vi "Get Active Timing Function.vi"(0 "Timing Functions in":refnum<class "ControllerData.lvclass">, 11 "error in (no error)":errorcluster) -> (4 "Timing Functions out":refnum<class "ControllerData.lvclass">, 6 "Function List":T1, 15 "error out":errorcluster)   [LabVIEW 2019, in "ControllerData.lvclass"]
uses:
  ControllerData.lvclass
  source code/LSL components/functions/functionsbase/functionbase.lvclass
  Function List.ctl
  D:/Pet Projects/LSL/source code/LSL components/functions/functionsbase/functionbase.lvclass
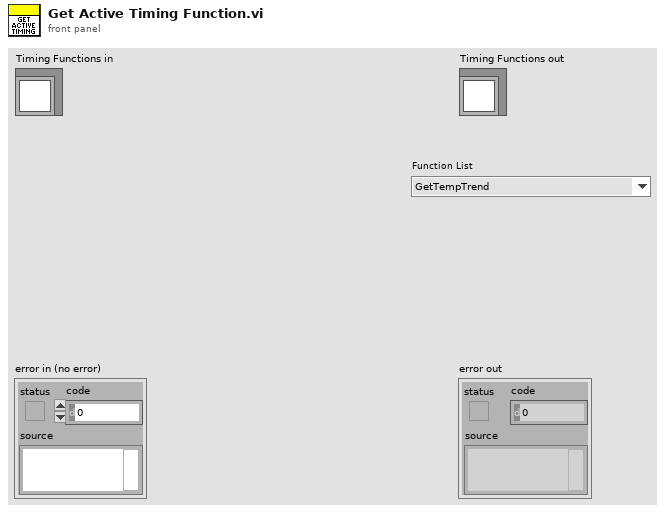
[diagram p1: front panel]
types:
  T1 = typedef "ControllerData.lvclass/Function List.ctl" = enum16{"GetTempTrend", "GetStatus"}
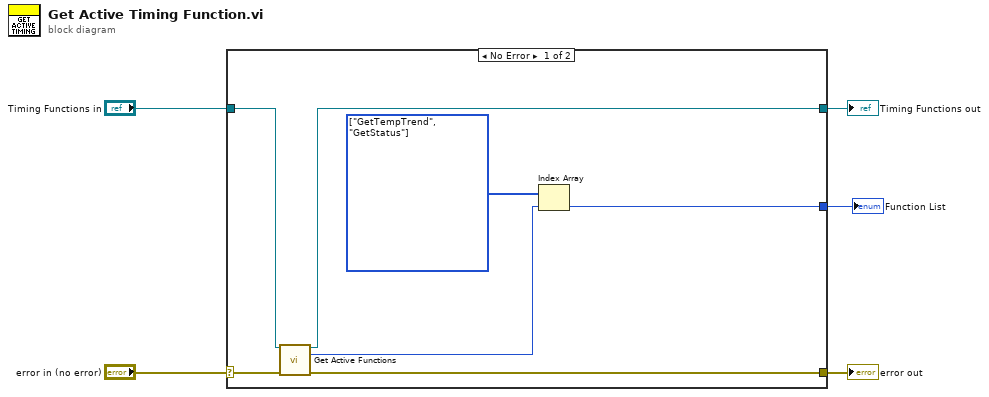
[diagram p0: block diagram]
diagram:
  n1 = case shown="No Error" "error in (no error)" {
    selector: "error in (no error)" -> [w12 w14]
    tunnel: [w11 w14] -> w4
    tunnel: [w9 w13] -> w2
    tunnel: "Timing Functions in" -> [w10 w13]
    tunnel: [w6 _] -> w1
    frame No Error {
      w8 = T1[] [enum."GetTempTrend", enum."GetStatus"] items=["GetTempTrend", "GetStatus"]
      n2 = call "Get Active Functions.vi"("functionbase in"=w10, "error in (no error)"=w12) -> ("functionbase out"=w9:refnum<class "ControllerData.lvclass">, "Syntax Index"=w7:i32, "error out"=w11:errorcluster)  [unwired: 11 in]
      n3 = Index Array(array=w8, index=w7) -> (element=w6:T1)
    }
    frame Error {
    }
  }
  "error out" <- w4
  "Timing Functions out" <- w2
  "Function List" <- w1
